vi "Set Boolean Text.vi"(8 "Error In":errorcluster, 9 "Mark Selected Errors As Read Button Reference":refnum<vi>, 10 "MCL Value":i32[](array[numeric])) -> (0 "Error Out":errorcluster)   [LabVIEW 2023, in "Error Manager.lvlib" / "Mark Selected Errors As Read Button.lvclass"]
doc: "This VI controls the Boolean Text of the button.\n If 0 or 1 MCL rows are selected, the boolean text is set to \"Mark Selected Error As Read\".\n If 2 or more rows are selected, the boolean text is set to \"Mark Selected Errors As Read\"."
uses:
  Mark Selected Errors As Read Button.lvclass
  Mark Selected Errors As Read Button.lvclass/Mark Selected Errors As Read Button.ctl
panel:
  out "Number of MCL rows selected":i32
  # "Development\nControls or indicators that are useful for development or testing, but which are not outputs of the VI."
  # "Input\nInputs to the VI"
  # "Output\nOutputs of the VI"
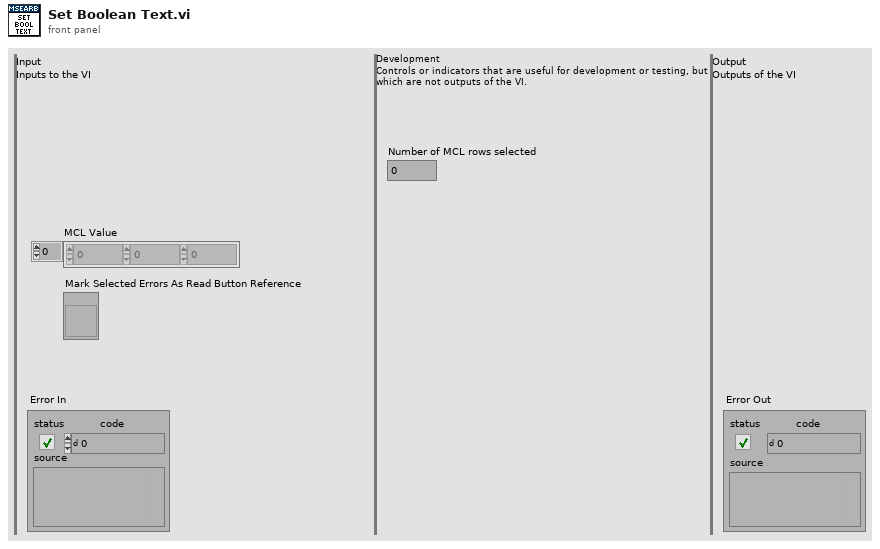
[diagram p1: front panel]
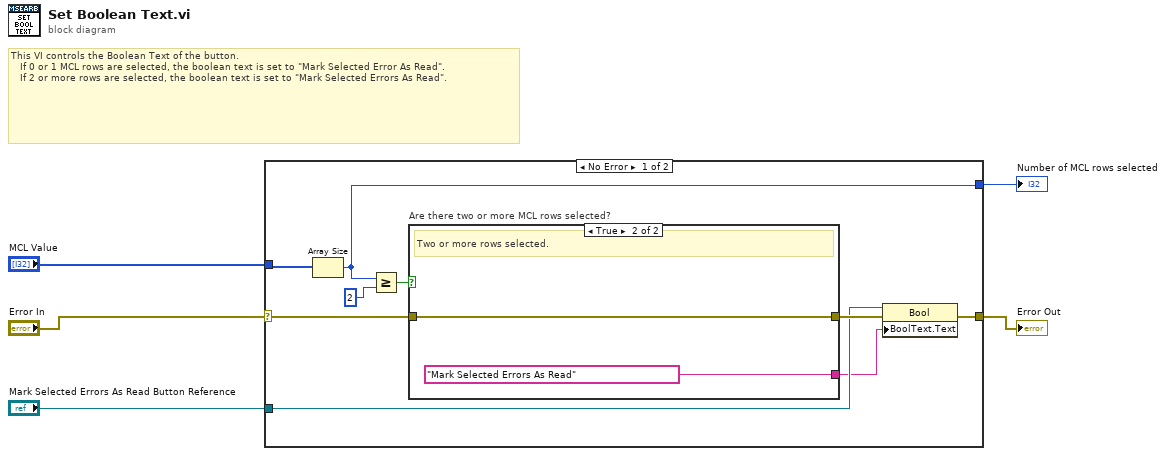
[diagram p0: block diagram]
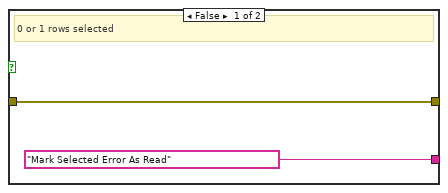
[diagram p2: hidden frame]
diagram:
  # "This VI controls the Boolean Text of the button.\n   If 0 or 1 MCL rows are selected, the boolean text is set to \"Mark Selected Error As Read\".\n   If 2 or more rows are selected, the boolean text is set to \"Mark Selected Errors As Read\"."
  n1 = case shown="No Error" "Error In" {
    selector: "Error In" -> [w14 w19]
    tunnel: [w9 w19] -> w4
    tunnel: "MCL Value" -> [w6 _]
    tunnel: [w10 _] -> w2
    tunnel: "Mark Selected Errors As Read Button Reference" -> [w8 _]
    frame No Error {
      n2 = Array Size(array=w6) -> (size(s)=w10:i32)
      n3 = Greater Or Equal?(x=w10, y=2) -> (x >= y?=w11:bool)
      n4 = case "Are there two or more MCL rows selected?" shown="True" w11 {
        tunnel: w14 -> [w16 w18]
        tunnel: [w16 w18] -> w12
        tunnel: ["Mark Selected Error As Read" ("Boolean Text.Text") "Mark Selected Errors As Read" ("Boolean Text.Text")] -> w7
        frame False {
          # "0 or 1 rows selected"
        }
        frame True {
          # "Two or more rows selected."
        }
      }
      n5 = property class="Bool"(reference=w8, error in=w12, "BoolText.Text"=w7) -> (error out=w9:errorcluster)  [unwired: 1 out]
    }
    frame Error {
    }
  }
  "Error Out" <- w4
  "Number of MCL rows selected" <- w2
